vi "ModInverseClarke (FXP).vi"(0 "a":fxp<+/-,32,12>, 1 "b":fxp<+/-,32,12>) -> (2 "A":fxp<+/-,32,12> format="%.24g", 3 "B":fxp<+/-,32,12> format="%.24g", 4 "C":fxp<+/-,32,12> format="%.24g")   [LabVIEW 2025]
uses:
  <vilib>/rvi/FXPMathLib/FxpMul/XNode/nifxpmath_Multiplier.xnode
  <vilib>/rvi/FXPMathLib/sim/FxpSim.dll
  <vilib>/rvi/FXPMathLib/FxpAdd/XNode/nifxpmath_Add.xnode
  <vilib>/rvi/FXPMathLib/FxpSub/XNode/nifxpmath_Sub.xnode
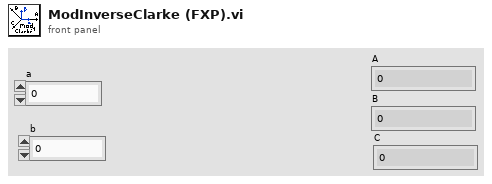
[diagram p1: front panel]
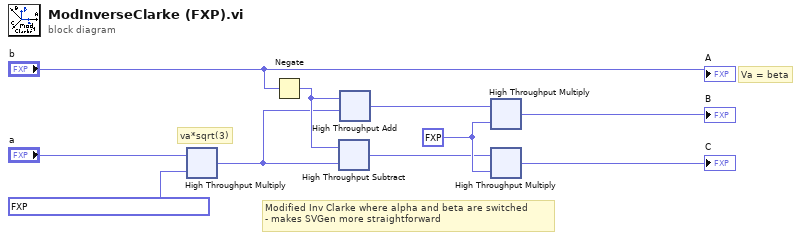
[diagram p0: block diagram]
diagram:
  w7 = fxp<+,1,0> 0.5
  # "Modified Inv Clarke where alpha and beta are switched\n- makes SVGen more straightforward"
  # "va*sqrt(3)"
  # "Va = beta"
  n1 = xnode "High Throughput Multiply"("a", fxp<+,32,1> 1.7320508076809347) -> (w8:fxp<+/-,32,13>)
  n2 = Negate(x="b") -> (-x=w10:fxp<+/-,33,13>)
  n3 = xnode "High Throughput Subtract"(w10, w8) -> (w6:fxp<+/-,37,17>)
  n4 = xnode "High Throughput Add"(w10, w8) -> (w5:fxp<+/-,37,17>)
  n5 = xnode "High Throughput Multiply"(w5, w7) -> (→"B":fxp<+/-,32,12>)
  n6 = xnode "High Throughput Multiply"(w6, w7) -> (→"C":fxp<+/-,32,12>)
  "A" <- "b"
